vi "Magnetic Sweep 1.4.vi"() -> ()   [LabVIEW 2011]
uses:
  <vilib>/Math Plots/3D Math Plots/3D Contour/3D Contour XCtrl/3D Contour.xctl
  <vilib>/Math Plots/3D Math Plots/3D Contour/3D Contour Datatype/Public/Plot Helper (Vector).vi
  <vilib>/Math Plots/3D Math Plots/3D Contour/3D Contour Datatype/3D Contour Datatype.lvclass
panel:
  in  "error out 4":errorcluster
  out "String":string="Persistent switch is not on"
  in  "Set parameter":bool
  out "status":string
  out "PID command":string
  out "setpoint command":string
  out "setpoint":dbl
  out "3D Contour \n(Ramp down)":refnum<class "3D Plot Datatype.lvclass">[](xcontrol)
  out "3D Contour\n(Ramp up)":refnum<class "3D Plot Datatype.lvclass">[](xcontrol)
  in  "stop":bool
  out "error out 3":errorcluster
  out "error out 2":errorcluster
  in  "Contour plot (ramp down)":path
  in  "Raw data (ramp down)":path
  out "Elapsed Time (s)":dbl
  out "Numeric":i32
  in  "error out":errorcluster
  out "Initial Temperature":string
  out "Zero field reached":bool
  out "Target field reached":bool
  in  "Upper limite":dbl
  in  "Temperature\nramping step":dbl
  in  "Heater range":i16(ring) items=["High", "Medium", "Low"]
  in  "D gain":dbl
  in  "I gain":dbl
  in  "P gain":dbl
  in  "Contour plot (ramp up)":path
  out "Time elapsed":string
  in  "Timer":bool caption="Reset"
  in  "date format":enum16{"short", "long", "abbreviated"}(ring)
  in  "Save":bool
  in  "Raw data (ramp  up)":path
  out "Temperature vs Time":cluster{dbl[], dbl[]}(graph)
  out "current time":timestamp
  out "Magnetic\nField":cluster{dbl[], dbl[]}(graph)
  out "Current Resistance":string
  out "Current Temperature":string
  out "Current Field":string
  out "Status":string
  in  "Field Sweep":bool
  in  "Magnetic field\nRamp rate":dbl
  in  "Traget Field":dbl
  out "Init Response":string
  in  "error in (no error)":errorcluster
  in  "IP Address":string
  in  "Ramp":bool
  in  "Update":bool
  in  "Ramp to Zero":bool
  in  "P Switch":bool
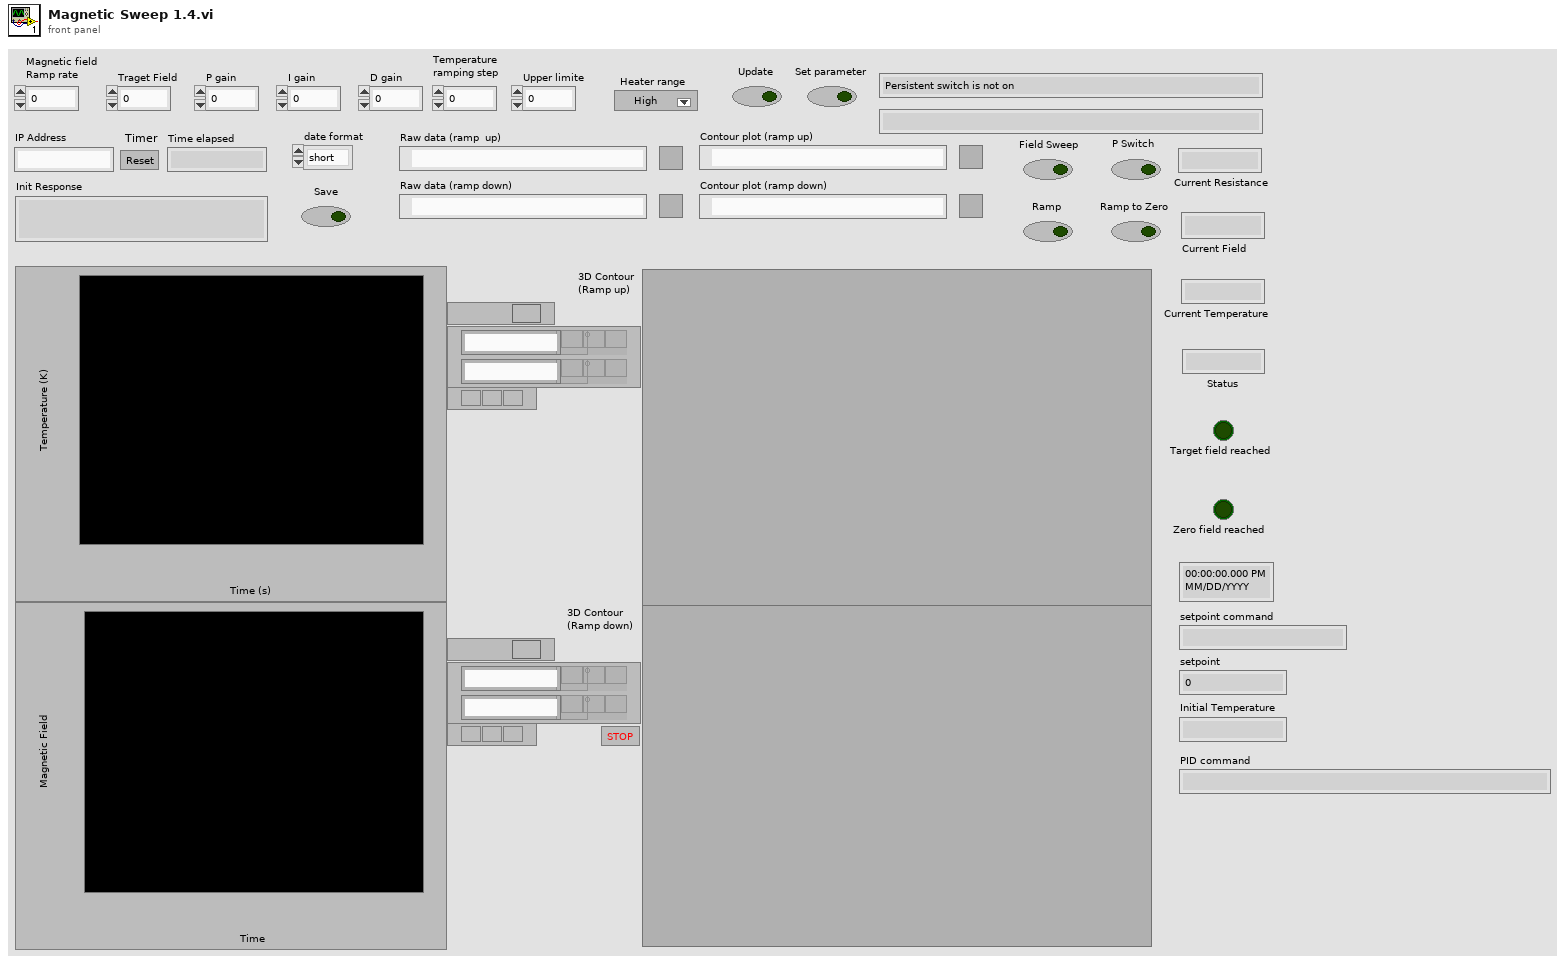
[diagram p1: front panel]
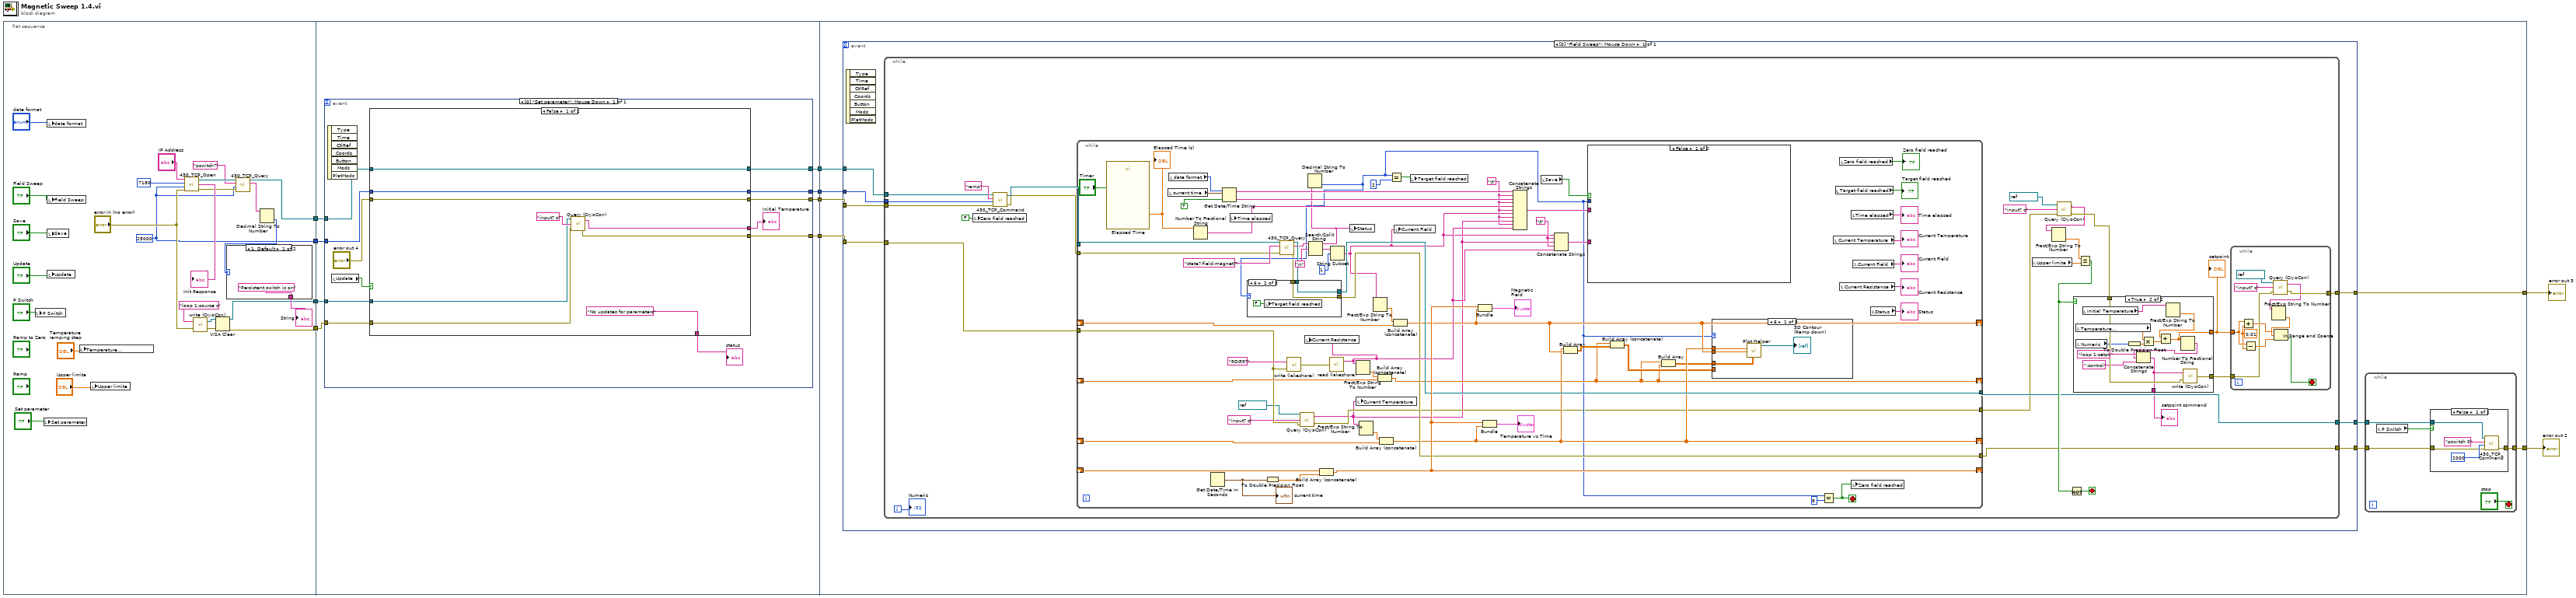
[diagram p0: block diagram]
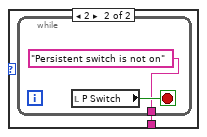
[diagram p2: hidden frame]
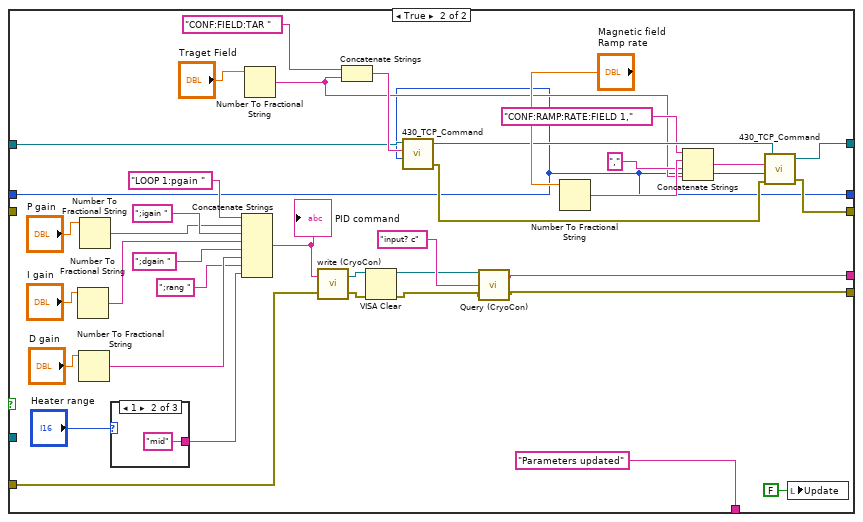
[diagram p3: hidden frame]
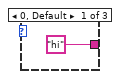
[diagram p4: hidden frame]
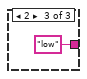
[diagram p5: hidden frame]
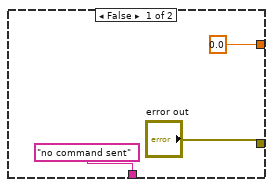
[diagram p7: hidden frame]
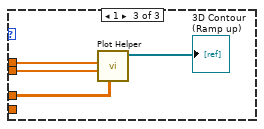
[diagram p9: hidden frame]
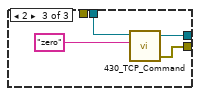
[diagram p11: hidden frame]
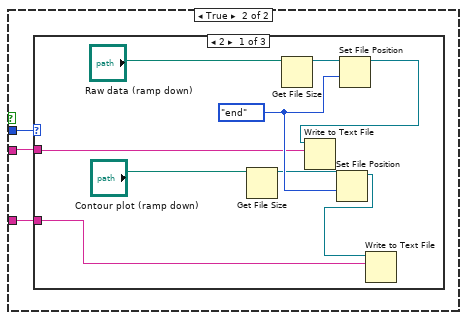
[diagram p12: hidden frame]
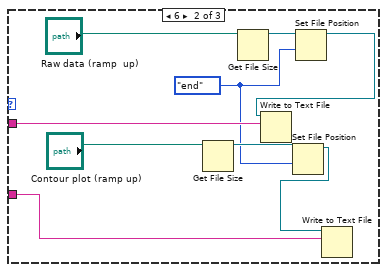
[diagram p13: hidden frame]
diagram:
  n1 = flat-sequence {
    tunnel: [w22] -> w10
    tunnel: [w11] -> w9
    tunnel: [w14] -> w8
    tunnel: [w12] -> w1
    tunnel: w10 -> [w47]
    tunnel: w9 -> [w46]
    tunnel: w8 -> [w45]
    tunnel: [w44] -> w7
    tunnel: [w43] -> w4
    tunnel: [w42] -> w3
    tunnel: [w41] -> w2
    tunnel: w1 -> [w40]
    tunnel: w7 -> [w117]
    tunnel: [w116] -> w6
    tunnel: [w114] -> w5
    tunnel: w4 -> [w112]
    tunnel: w3 -> [w111]
    tunnel: w2 -> [w110]
    frame #0 {
      w11 = 25000 ("Timeout")
      n2 = local write "P Switch"("P Switch") -> ()
      n3 = local write "Set parameter"("Set parameter") -> ()
      n4 = local write "date format"("date format") -> ()
      n5 = local write "Field Sweep"("Field Sweep") -> ()
      n6 = local write "Save"("Save") -> ()
      n7 = local write "Update"("Update") -> ()
      n8 = local write "Temperature\nramping step"("Temperature\nramping step") -> ()
      n9 = local write "Upper limite"("Upper limite") -> ()
      n10 = call "430_TCP_Open.vi"("IP Address"="IP Address", "TCP Port"=7180, "timeout ms (2000)"=w11, "error in (no error)"="error in (no error)") -> ("connection ID"=w23:refnum<k5>, "Init Response"=→"Init Response":string, "error out"=w21:errorcluster)  [unwired: 2 in]
      n11 = call "write (CryoCon).vi"("error in (no error)"="error in (no error)", "write buffer"="loop 1:source c") -> ("error out"=w16:errorcluster, "VISA resource name out"=w15:refnum<visa-resource-name>)
      n12 = VISA Clear(VISA resource name=w15, error in (no error)=w16) -> (VISA resource name out=w12:refnum<visa-resource-name>, error out=w14:errorcluster)
      n13 = call "430_TCP_Query.vi"("error in (no error)"=w21, "Timeout"=w11, "Command"="pswitch?", "connection ID"=w23) -> ("Response"=w19:string, "connection ID out"=w22:refnum<k5>)  [unwired: 3 in, 3 out]
      n14 = Decimal String To Number(string=w19) -> (number=w18:i32)  [unwired: 2 in, 1 out]
      n15 = case shown="1, Default" w18 {
        tunnel: ["Persistent switch is on" w37] -> w13
        frame 1, Default {
        }
        frame 2 {
          n16 = while {
            tunnel: ["Persistent switch is not on"] -> w37
            stop <- w39 stop-if-true
            n17 = local read "P Switch"() -> (w39:bool)
          }
        }
      }
      "String" <- w13
    }
    frame #1 {
      n18 = event shown="[0] \"Set parameter\": Mouse Down" {
        selector: _ -> [_]
        dyn-events: _ -> [_]
        timeout: _ -> [_]
        tunnel: w47 -> [w59]
        tunnel: w46 -> [w58]
        tunnel: w45 -> [w57]
        tunnel: [w56] -> w44
        tunnel: [w55] -> w43
        tunnel: [w54] -> w42
        tunnel: [w53] -> w41
        tunnel: w40 -> [w49]
        event "Set parameter": Mouse Down {
          n19 = event-data() -> ()  [unwired: 1 in, 7 out]
          n20 = local read "Update"() -> (w50:bool)
          n21 = case shown="False" w50 {
            tunnel: w59 -> [w66 w104]
            tunnel: w58 -> [w67 w76]
            tunnel: w57 -> [w61 w83]
            tunnel: [w62 w69] -> w56
            tunnel: ["No updates for parameters" ("String") "Parameters updated" ("String")] -> w52
            tunnel: [w60 w78] -> w55
            tunnel: [w66 w77] -> w54
            tunnel: [w67 w76] -> w53
            tunnel: [w63 w70] -> w51
            tunnel: w49 -> [w64 _]
            tunnel: "error out 4" -> [w60 _]
            frame False {
              n22 = call "Query (CryoCon).vi"("error in (no error)"=w61, "write buffer"="input? c", "VISA resource name 2"=w64) -> ("error out"=w62:errorcluster, "read buffer"=w63:string)
            }
            frame True {
              n23 = Number To Fractional String(number="I gain") -> (F-format string=w87:string)  [unwired: 3 in]
              n24 = Number To Fractional String(number="D gain") -> (F-format string=w85:string)  [unwired: 3 in]
              n25 = Number To Fractional String(number="P gain") -> (F-format string=w88:string)  [unwired: 3 in]
              n26 = case shown="1" "Heater range" {
                tunnel: ["hi" "mid" "low"] -> w80
                frame 0, Default {
                }
                frame 1 {
                }
                frame 2 {
                }
              }
              n27 = Concatenate Strings("LOOP 1:pgain " ("write buffer"), w88, ";igain " ("string"), w87, ";dgain " ("string"), w85, ";rang " ("string"), w80) -> (w84:string)
              "PID command" <- w84
              n28 = Number To Fractional String(number="Traget Field") -> (F-format string=w94:string)  [unwired: 3 in]
              n29 = call "write (CryoCon).vi"("error in (no error)"=w83, "write buffer"=w84) -> ("error out"=w75:errorcluster, "VISA resource name out"=w74:refnum<visa-resource-name>)
              n30 = Concatenate Strings("CONF:FIELD:TAR ", w94) -> (w105:string)
              n31 = VISA Clear(VISA resource name=w74, error in (no error)=w75) -> (VISA resource name out=w71:refnum<visa-resource-name>, error out=w72:errorcluster)
              n32 = call "430_TCP_Command.vi"("Timeout"=w76, "Command"=w105, "connection ID"=w104) -> ("error out"=w103:errorcluster, "connection ID out"=w99:refnum<k5>)  [unwired: 1 in, 1 out]
              n33 = call "Query (CryoCon).vi"("error in (no error)"=w72, "write buffer"="input? c", "VISA resource name 2"=w71) -> ("error out"=w69:errorcluster, "read buffer"=w70:string)
              n34 = Number To Fractional String(number="Magnetic field\nRamp rate") -> (F-format string=w97:string)  [unwired: 3 in]
              n35 = Concatenate Strings("CONF:RAMP:RATE:FIELD 1," ("string"), w97, "," ("string"), w94) -> (w100:string)
              n36 = call "430_TCP_Command.vi"("error in (no error)"=w103, "Timeout"=w76, "Command"=w100, "connection ID"=w99) -> ("error out"=w78:errorcluster, "connection ID out"=w77:refnum<k5>)  [unwired: 1 out]
              n37 = local write "Update"(FALSE ("Update")) -> ()
            }
          }
          "Initial Temperature" <- w51
          "status" <- w52
        }
      }
    }
    frame #2 {
      n38 = event shown="[0] \"Field Sweep\": Mouse Down" {
        selector: _ -> [_]
        dyn-events: _ -> [_]
        timeout: _ -> [_]
        tunnel: w117 -> [w135]
        tunnel: [w134] -> w116
        tunnel: [w133] -> w115
        tunnel: [w132] -> w113
        tunnel: w112 -> [w131]
        tunnel: w111 -> [w130]
        tunnel: w110 -> [w129]
        event "Field Sweep": Mouse Down {
          n39 = event-data() -> ()  [unwired: 1 in, 7 out]
          n40 = while {
            tunnel: w135 -> [w157]
            tunnel: [w147] -> w134
            tunnel: [w146] -> w133
            tunnel: [w145] -> w132
            tunnel: w131 -> [w143]
            tunnel: w130 -> [w142]
            tunnel: w129 -> [w141]
            i -> [w154]
            stop <- w149 stop-if-true
            n41 = local write "Zero field reached"(FALSE ("Zero field reached")) -> ()
            n42 = call "430_TCP_Command.vi"("error in (no error)"=w143, "Timeout"=w141, "Command"="ramp", "connection ID"=w142) -> ("error out"=w159:errorcluster, "connection ID out"=w158:refnum<k5>)  [unwired: 1 out]
            n43 = while {
              shift-right: [w197] -> _
              shift-left: _ -> [w244]
              shift-right: [w198] -> _
              shift-left: _ -> [w249]
              shift-right: [w194] -> _
              shift-left: _ -> [w246]
              shift-right: [w239] -> _
              shift-left: _ -> [w240]
              tunnel: w159 -> [w228]
              tunnel: w158 -> [w227]
              tunnel: w157 -> [w191]
              tunnel: [w190] -> w139
              tunnel: [w207] -> w146
              tunnel: [w206] -> w145
              stop <- w210 stop-if-true
              w232 = "\t"
              w233 = "\t"
              n44 = call "Elapsed Time"("Reset"="Timer") -> ("Elapsed Time (s)"=w221:dbl)  [unwired: 11 in, 7 out]
              "Elapsed Time (s)" <- w221
              n45 = local read "current time"() -> (w230:timestamp)
              n46 = local read "date format"() -> (w223:enum16{"short", "long", "abbreviated"})
              n47 = Number To Fractional String(number=w221) -> (F-format string=w225:string)  [unwired: 3 in]
              n48 = Get Date/Time In Seconds() -> (seconds since 1Jan1904=w220:timestamp)
              "current time" <- w220
              n49 = Get Date/Time String(date format (0)=w223, seconds (now)=w230, want seconds? (F)=TRUE) -> (date string=w235:string, time string=w234:string)
              n50 = local write "Time elapsed"(w225) -> ()
              n51 = To Double Precision Float(number=w220) -> (double precision float=w241:dbl)
              n52 = call "430_TCP_Query.vi"("error in (no error)"=w228, "Command"="state?;field:magnet?", "connection ID"=w227) -> ("error out"=w192:errorcluster, "Response"=w205:string, "connection ID out"=w209:refnum<k5>)  [unwired: 4 in, 2 out]
              n53 = call "write (lakeshore).vi"("error in (no error)"=w191, "write buffer"="RDGR?") -> ("error out"=w248:errorcluster)
              n54 = call "Query (CryoCon).vi"("error in (no error)"=w191, "write buffer"="input? c", "VISA resource name 2"=refnum<visa-resource-name> "COM3") -> ("error out"=w190:errorcluster, "read buffer"=w189:string)
              n55 = Search/Split String(string=w205, search string/char (-)="\n") -> (substring before match=w204:string, match + rest of string=w203:string)  [unwired: 1 in, 1 out]
              n56 = Decimal String To Number(string=w204) -> (number=w193:i32)  [unwired: 2 in, 1 out]
              n57 = case shown="6" w193 {
                tunnel: [w259 w261 w266] -> w206
                tunnel: w209 -> [w260 w263 w265]
                tunnel: [w260 w263 w264] -> w207
                tunnel: w192 -> [w259 w261 _]
                frame 0, Default {
                }
                frame 6 {
                  n58 = local write "Target field reached"(FALSE ("Target field reached")) -> ()
                }
                frame 2 {
                  n59 = call "430_TCP_Command.vi"("Command"="zero", "connection ID"=w265) -> ("error out"=w266:errorcluster, "connection ID out"=w264:refnum<k5>)  [unwired: 2 in, 1 out]
                }
              }
              n60 = Build Array (concatenate)(w240, w241) -> (w239:dbl[])
              n61 = call "read (lakeshore).vi"("error in (no error)"=w248) -> ("read buffer"=w224:string)  [unwired: 1 out]
              n62 = local write "Current Resistance"(w224) -> ()
              n63 = String Subset(string=w203, offset (0)=1) -> (substring=w201:string)  [unwired: 1 in]
              n64 = local write "Status"(w204) -> ()
              n65 = Fract/Exp String To Number(string=w224) -> (number=w242:dbl)  [unwired: 3 in, 1 out]
              n66 = local write "Current Temperature"(w189) -> ()
              n67 = Fract/Exp String To Number(string=w189) -> (number=w243:dbl)  [unwired: 3 in, 1 out]
              n68 = Fract/Exp String To Number(string=w201) -> (number=w245:dbl)  [unwired: 3 in, 1 out]
              n69 = Build Array (concatenate)(w242, w246) -> (w194:dbl[])
              n70 = Build Array (concatenate)(w243, w249) -> (w198:dbl[])
              n71 = Equal?(x=w193, y=2) -> (x = y?=w226:bool)
              n72 = Build Array (concatenate)(w245, w244) -> (w197:dbl[])
              n73 = local write "Current Field"(w201) -> ()
              n74 = local write "Target field reached"(w226) -> ()
              n75 = Bundle(w239, w197) -> (→"Magnetic\nField":cluster{dbl[], dbl[]})  [unwired: 1 in]
              n76 = Bundle(w239, w198) -> (→"Temperature vs Time":cluster{dbl[], dbl[]})  [unwired: 1 in]
              n77 = Concatenate Strings(w235, w233, w234, w233, w225, w233, w201, w233, w189, w233, w224) -> (w238:string)
              n78 = local read "Save"() -> (w219:bool)
              n79 = Concatenate Strings(w201, w232, w189, w232, w224) -> (w231:string)
              n80 = Build Array(w198, w197) -> (w208:dbl[][])
              n81 = case shown="False" w219 {
                tunnel: w238 -> [_ w270]
                tunnel: w231 -> [_ w269]
                tunnel: w193 -> [_ w268]
                frame False {
                }
                frame True {
                  n82 = case shown="2" w268 {
                    tunnel: w270 -> [w272 w288 _]
                    tunnel: w269 -> [w271 w282 _]
                    frame 2 {
                      w278 = enum16{"start", "end", "current"}."end" ("from (0:start)")
                      n83 = Get File Size(file="Contour plot (ramp down)") -> (refnum out=w277:refnum<file>)  [unwired: 1 in, 2 out]
                      n84 = Get File Size(file="Raw data (ramp down)") -> (refnum out=w274:refnum<file>)  [unwired: 1 in, 2 out]
                      n85 = Set File Position(refnum=w277, from (0:start)=w278) -> (refnum out=w279:refnum<file>)  [unwired: 2 in, 1 out]
                      n86 = Set File Position(refnum=w274, from (0:start)=w278) -> (refnum out=w275:refnum<file>)  [unwired: 2 in, 1 out]
                      n87 = Write to Text File(file (use dialog)=w275, text=w272) -> ()  [unwired: 2 in, 3 out]
                      n88 = Write to Text File(file (use dialog)=w279, text=w271) -> ()  [unwired: 2 in, 3 out]
                    }
                    frame 6 {
                      w281 = enum16{"start", "end", "current"}."end" ("from (0:start)")
                      n89 = Get File Size(file="Contour plot (ramp up)") -> (refnum out=w283:refnum<file>)  [unwired: 1 in, 2 out]
                      n90 = Get File Size(file="Raw data (ramp  up)") -> (refnum out=w286:refnum<file>)  [unwired: 1 in, 2 out]
                      n91 = Set File Position(refnum=w283, from (0:start)=w281) -> (refnum out=w280:refnum<file>)  [unwired: 2 in, 1 out]
                      n92 = Set File Position(refnum=w286, from (0:start)=w281) -> (refnum out=w285:refnum<file>)  [unwired: 2 in, 1 out]
                      n93 = Write to Text File(file (use dialog)=w285, text=w288) -> ()  [unwired: 2 in, 3 out]
                      n94 = Write to Text File(file (use dialog)=w280, text=w282) -> ()  [unwired: 2 in, 3 out]
                    }
                    frame Default {
                    }
                  }
                }
              }
              n95 = Build Array (concatenate)(w194, w208) -> (w195:dbl[][])
              n96 = Build Array(w194, w194) -> (w196:dbl[][])
              n97 = case shown="6" w193 {
                tunnel: w198 -> [w253 _ w257]
                tunnel: w197 -> [w252 _ w256]
                tunnel: w196 -> [w251 _ w255]
                tunnel: w195 -> [_ _ _]
                frame 6 {
                  n98 = call-poly <vilib>:"Plot Helper.vi"("z matrix"=w251, "y vector"=w252, "x vector"=w253) -> ("3D Plot lvclass Array out"=→"3D Contour \n(Ramp down)":refnum<class "3D Plot Datatype.lvclass">[])  [unwired: 3 in, 5 out]
                }
                frame 0, Default {
                }
                frame 1 {
                  n99 = call-poly <vilib>:"Plot Helper.vi"("z matrix"=w255, "y vector"=w256, "x vector"=w257) -> ("3D Plot lvclass Array out"=→"3D Contour\n(Ramp up)":refnum<class "3D Plot Datatype.lvclass">[])  [unwired: 3 in, 5 out]
                }
              }
              n100 = Equal?(x=w193, y=8) -> (x = y?=w210:bool)
              n101 = local read "Current Temperature"() -> (→"Current Temperature":string)
              n102 = local read "Target field reached"() -> (→"Target field reached":bool)
              n103 = local read "Zero field reached"() -> (→"Zero field reached":bool)
              n104 = local read "Current Resistance"() -> (→"Current Resistance":string)
              n105 = local read "Time elapsed"() -> (→"Time elapsed":string)
              n106 = local write "Zero field reached"(w210) -> ()
              n107 = local read "Current Field"() -> (→"Current Field":string)
              n108 = local read "Status"() -> (→"Status":string)
            }
            n109 = local read "Upper limite"() -> (w151:dbl)
            n110 = call "Query (CryoCon).vi"("error in (no error)"=w139, "write buffer"="input? c", "VISA resource name 2"=refnum<visa-resource-name> "COM3") -> ("error out"=w138:errorcluster, "read buffer"=w137:string)
            n111 = Fract/Exp String To Number(string=w137) -> (number=w150:dbl)  [unwired: 3 in, 1 out]
            n112 = Less Or Equal?(x=w150, y=w151) -> (x <= y?=w148:bool)
            n113 = Not(x=w148) -> (.not. x?=w149:bool)
            n114 = case shown="True" w148 {
              tunnel: w138 -> [_ w184]
              tunnel: ["error out" w181] -> w156
              tunnel: [0.0 w180] -> w155
              tunnel: ["no command sent" w174] -> w144
              frame False {
              }
              frame True {
                n115 = local read "Temperature\nramping step"() -> (w178:dbl)
                n116 = local read "Numeric"() -> (w176:i32)
                n117 = local read "Initial Temperature"() -> (w183:string)
                n118 = To Double Precision Float(number=w176) -> (double precision float=w177:dbl)
                n119 = Multiply(x=w178, y=w177) -> (x*y=w179:dbl)
                n120 = Fract/Exp String To Number(string=w183) -> (number=w182:dbl)  [unwired: 3 in, 1 out]
                n121 = Add(x=w182, y=w179) -> (x+y=w180:dbl)
                n122 = Number To Fractional String(number=w180) -> (F-format string=w185:string)  [unwired: 3 in]
                n123 = Concatenate Strings("loop 1:setpt " ("write buffer"), w185, ";control" ("string")) -> (w174:string)
                n124 = call "write (CryoCon).vi"("error in (no error)"=w184, "write buffer"=w174) -> ("error out"=w181:errorcluster)  [unwired: 1 out]
              }
            }
            "setpoint" <- w155
            "setpoint command" <- w144
            n125 = while {
              tunnel: w156 -> [w162]
              tunnel: w155 -> [w169]
              tunnel: [w161] -> w147
              stop <- w165 stop-if-true
              w166 = 0.01 ("y")
              n126 = Add(x=w169, y=w166) -> (x+y=w168:dbl)
              n127 = Subtract(x=w169, y=w166) -> (x-y=w167:dbl)
              n128 = call "Query (CryoCon).vi"("error in (no error)"=w162, "write buffer"="input? c", "VISA resource name 2"=refnum<visa-resource-name> "COM3") -> ("error out"=w161:errorcluster, "read buffer"=w160:string)
              n129 = Fract/Exp String To Number(string=w160) -> (number=w170:dbl)  [unwired: 3 in, 1 out]
              n130 = In Range and Coerce(upper limit=w168, x=w170, lower limit=w167) -> (In Range?=w165:bool)  [unwired: 1 out]
            }
            "Numeric" <- w154
          }
        }
      }
      n131 = while {
        tunnel: w115 -> [w122]
        tunnel: [w120] -> w114
        tunnel: w113 -> [w119]
        stop <- "stop" stop-if-true
        n132 = local read "P Switch"() -> (w121:bool)
        n133 = case shown="False" w121 {
          tunnel: w122 -> [w126 _]
          tunnel: [w124 w128] -> w120
          tunnel: w119 -> [w123 w128]
          frame False {
            n134 = call "430_TCP_Command.vi"("error in (no error)"=w123, "Timeout"=2000, "Command"="pswitch 0", "connection ID"=w126) -> ("error out"=w124:errorcluster)  [unwired: 2 out]
          }
          frame True {
          }
        }
      }
    }
  }
  "error out 2" <- w5
  "error out 3" <- w6
